vi "tls http parse function.vi"(10 "data in":string, 11 "application request in":T1) -> (2 "error":bool, 3 "application request out":T1)   [LabVIEW 2016, in "Basic HTTPS server.lvclass"]
uses:
  Basic HTTPS server.lvclass
  http request.ctl
  http method.ctl
  HTTP headers/http header data.ctl
  HTTP headers/http headers.lvlib
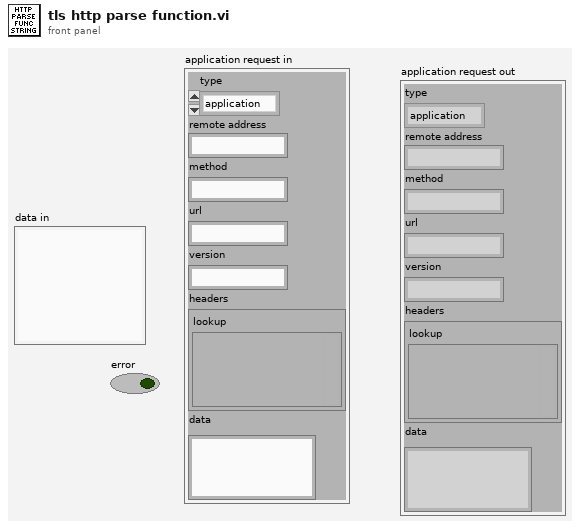
[diagram p1: front panel]
types:
  T1 = typedef "Basic HTTPS server.lvclass/http request.ctl" = cluster{"type":T2, "remote address":string, "method":string, "url":string, "version":string, "headers":T3, "data":string}
  T2 = typedef "Basic HTTPS server.lvclass/http method.ctl" = enum16{"application", "error", "upgrade"}
  T3 = typedef "http headers.lvlib/http header data.ctl" = cluster{"lookup":variant}
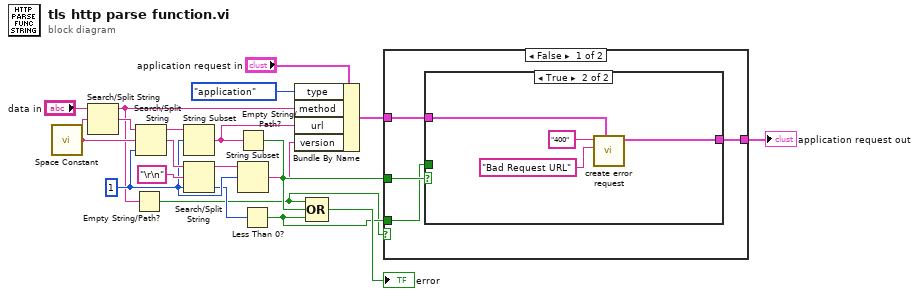
[diagram p0: block diagram]
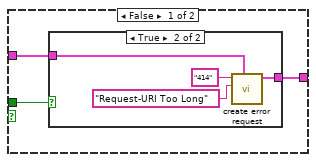
[diagram p2: hidden frame]
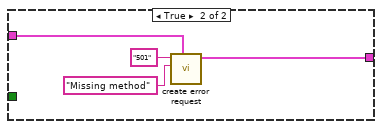
[diagram p4: hidden frame]
diagram:
  w9 = 1 ("offset (0)")
  n1 = call <vilib>:"Space Constant.vi"() -> ("String"=w15:string)
  n2 = Search/Split String(string="data in", search string/char (-)=w15) -> (substring before match=w4:string, match + rest of string=w16:string)  [unwired: 1 in, 1 out]
  n3 = Empty String/Path?(string/path=w4) -> (empty?=w3:bool)
  n4 = Search/Split String(string=w16, search string/char (-)=w15, offset (0)=w9) -> (substring before match=w14:string, match + rest of string=w12:string)  [unwired: 1 out]
  n5 = String Subset(string=w14, offset (0)=w9) -> (substring=w13:string)  [unwired: 1 in]
  n6 = Search/Split String(string=w12, search string/char (-)="\r\n", offset (0)=w9) -> (substring before match=w10:string, offset of match=w7:i32)  [unwired: 1 out]
  n7 = Empty String/Path?(string/path=w13) -> (empty?=w18:bool)
  n8 = String Subset(string=w10, offset (0)=w9) -> (substring=w8:string)  [unwired: 1 in]
  n9 = Less Than 0?(x=w7) -> (x < 0?=w6:bool)
  n10 = Bundle By Name(cluster="application request in", "type"=http_method."application", "method"=w4, "url"=w13, "version"=w8) -> (w2:T1)
  n11 = Compound Arithmetic op=OR(w3, w18, w6) -> (→"error":bool)
  n12 = case shown="False" w3 {
    tunnel: w18 -> [w24 _]
    tunnel: w6 -> [w23 _]
    tunnel: w2 -> [w22 w38]
    tunnel: [w21 w37] -> w1
    frame False {
      n13 = case shown="True" w24 {
        tunnel: w23 -> [w27 _]
        tunnel: w22 -> [w26 w34]
        tunnel: [w25 w33] -> w21
        frame False {
          n14 = case shown="True" w27 {
            tunnel: w26 -> [w28 w30]
            tunnel: [w28 w29] -> w25
            frame False {
            }
            frame True {
              n15 = call "create error request.vi"("incoming request"=w30, "reason"="Request-URI Too Long" ("status string"), "code"="414") -> ("element"=w29:T1)  [unwired: 8 in]
            }
          }
        }
        frame True {
          n16 = call "create error request.vi"("incoming request"=w34, "reason"="Bad Request URL" ("data"), "code"="400" ("method")) -> ("element"=w33:T1)  [unwired: 8 in]
        }
      }
    }
    frame True {
      n17 = call "create error request.vi"("incoming request"=w38, "reason"="Missing method" ("data"), "code"="501" ("method")) -> ("element"=w37:T1)  [unwired: 8 in]
    }
  }
  "application request out" <- w1
